vi "Calculate capture moves.vi"(7 "Position in":refnum<class "Position.lvclass">, 11 "Source":T1) -> (3 "Capture moves":refnum<class "Move.lvclass">[](array[class]))   [LabVIEW 2016, in "Chesslib.lvlib" / "Pawn.lvclass"]
uses:
  Pawn.lvclass
  Position/Position.lvclass
  Moves/Move/Move.lvclass
  typedef/Square.ctl
  typedef/File.ctl
  typedef/Rank.ctl
  typedef/Neighbor.ctl
  Piece/Piece.lvclass/Piece.ctl
  Chesslib.lvlib
  Piece/Piece.lvclass
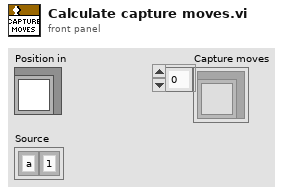
[diagram p1: front panel]
types:
  T1 = typedef "Chesslib.lvlib/Square.ctl" = cluster{"File":T2, "Rank":T3}
  T2 = typedef "Chesslib.lvlib/File.ctl" = enum8{"a", "b", "c", "d", "e", "f", "g", "h"}
  T3 = typedef "Chesslib.lvlib/Rank.ctl" = enum8{"1", "2", "3", "4", "5", "6", "7", "8"}
  T4 = typedef "Chesslib.lvlib/Color.ctl" = enum16{"White", "Black"}
  T5 = typedef "Chesslib.lvlib/Neighbor.ctl" = enum16{"N", "NW", "W", "SW", "S", "SE", "E", "NE", "vector"}
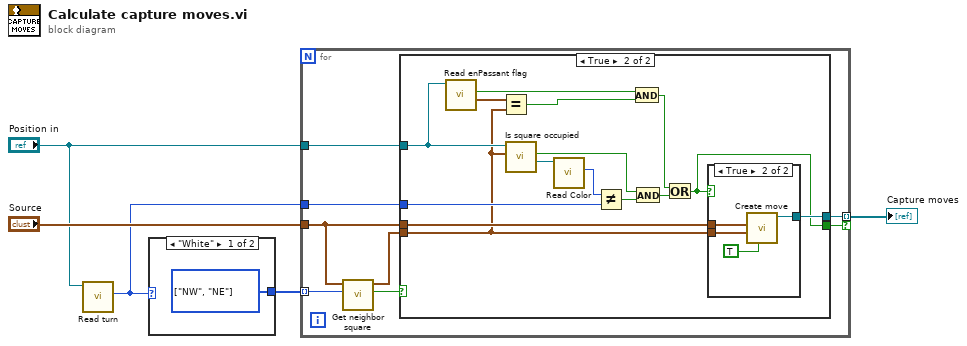
[diagram p0: block diagram]
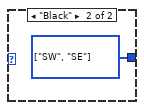
[diagram p4: hidden frame]
diagram:
  n1 = call "Read turn.vi"("Position in"="Position in") -> ("Turn"=w2:T4)  [unwired: 9 in, 1 out]
  n2 = case shown="\"White\"" w2 {
    tunnel: [w6 w7] -> w4
    frame "White" {
      w6 = T5[] [enum."NW", enum."NE"] items=["N", "NW", "W", "SW", "S", "SE", "E", "NE", "vector"] ("Neighbor (vector)")
    }
    frame "Black" {
      w7 = T5[] [enum."SW", enum."SE"] items=["N", "NW", "W", "SW", "S", "SE", "E", "NE", "vector"] ("Neighbor (vector)")
    }
  }
  n3 = for {
    tunnel: "Source" -> [w14]
    tunnel: "Position in" -> [w10]
    tunnel: w4 -> [w15] mode=indexing
    tunnel: [w13] -> w3 mode=indexing if=w11
    tunnel: w2 -> [w12]
    n4 = call "Get neighbor square.vi"("Neighbor (vector)"=w15, "Square in"=w14) -> ("Valid"=w8:bool, "Square out"=w9:T1)  [unwired: 7 in, 1 out]
    n5 = case shown="True" w8 {
      tunnel: w14 -> [_ w30]
      tunnel: [_ w29] -> w13
      tunnel: w12 -> [_ w28]
      tunnel: [_ w18] -> w11
      tunnel: w10 -> [_ w24]
      tunnel: w9 -> [_ w22]
      frame False {
      }
      frame True {
        n6 = call "Read enPassant flag.vi"("Position in"=w24) -> ("en Passant target"=w23:T1, "en Passant allowed?"=w21:bool)  [unwired: 8 in, 1 out]
        n7 = Equal?(x=w23, y=w22) -> (x = y?=w19:bool)
        n8 = call "Is square occupied.vi"("Square"=w22, "Position in"=w24) -> ("Piece"=w17:refnum<class "Piece.lvclass">, "Occupied"=w16:bool)  [unwired: 6 in, 2 out]
        n9 = call "Read Color.vi"("Piece in"=w17) -> ("Color"=w27:T4)  [unwired: 10 in]
        n10 = Not Equal?(x=w27, y=w28) -> (x != y?=w26:bool)
        n11 = And(x=w21, y=w19) -> (x .and. y?=w20:bool)
        n12 = And(x=w16, y=w26) -> (x .and. y?=w25:bool)
        n13 = Or(x=w20, y=w25) -> (x .or. y?=w18:bool)
        n14 = case shown="True" w18 {
          tunnel: w30 -> [_ w33]
          tunnel: w22 -> [_ w32]
          tunnel: [_ w31] -> w29
          frame False {
          }
          frame True {
            n15 = call "Create move.vi"("Pawn move (F)"=TRUE, "Destination"=w32, "Source"=w33) -> ("Move out"=w31:refnum<class "Move.lvclass">)  [unwired: 8 in]
          }
        }
      }
    }
  }
  "Capture moves" <- w3
